vi "CheckConnection.vi"(8 "error in (no error)":errorcluster, 11 "VISA Refnum in":refnum<visa-resource-name>) -> (0 "error out":errorcluster, 3 "Communication succeded?":bool)   [LabVIEW 2018]
doc: "Sends Set Target Command to Maestro channel 5 with control value and checks if value returned after sending Get Position command will correspond, if it does then communication succeded."
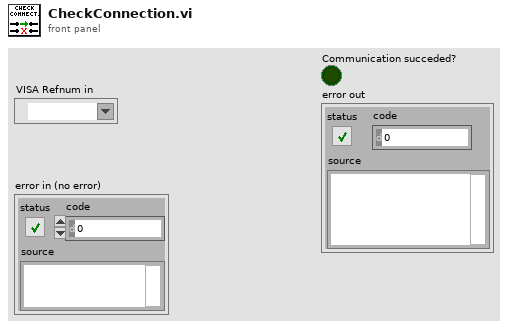
[diagram p1: front panel]
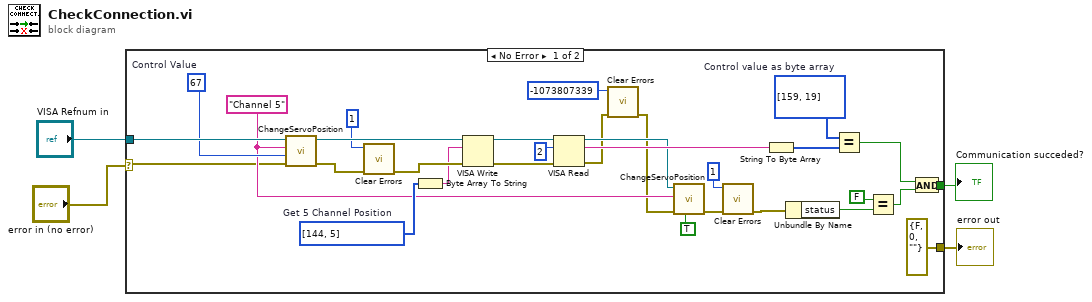
[diagram p0: block diagram]
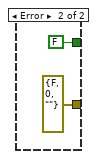
[diagram p2: hidden frame]
diagram:
  n1 = case shown="No Error" "error in (no error)" {
    selector: "error in (no error)" -> [w6 _]
    tunnel: [w32 FALSE] -> w4
    tunnel: "VISA Refnum in" -> [w29 _]
    tunnel: [errorcluster {"status"=FALSE, "code"=0, "source"=""} ("error out") errorcluster {"status"=FALSE, "code"=0, "source"=""} ("error out")] -> w2
    frame No Error {
      w21 = u8[] [144, 5]  # Get 5 Channel Position
      w15 = "Channel 5" ("Label.Text")
      w28 = i16 67  # Control Value
      w16 = u8[] [159, 19]  # Control value as byte array
      n2 = call "ChangeServoPosition.vi"("error in (no error)"=w6, "Value"=w28, "Label.Text"=w15, "VISA Refnum in"=w29) -> ("error out"=w27:errorcluster, "VISA resource name out"=w26:refnum<visa-resource-name>)  [unwired: 6 in]
      n3 = call <vilib>:"Clear Errors.vi"("error in (no error)"=w27, "specific error code to clear (0: all)"=1) -> ("error out"=w25:errorcluster)  [unwired: 4 in, 1 out]
      n4 = Byte Array To String(unsigned byte array=w21) -> (string=w22:string)
      n5 = VISA Write(VISA resource name=w26, write buffer=w22, error in (no error)=w25) -> (VISA resource name out=w24:refnum<visa-resource-name>, error out=w23:errorcluster)  [unwired: 1 out]
      n6 = VISA Read(VISA resource name=w24, byte count=u32 2, error in (no error)=w23) -> (VISA resource name out=w14:refnum<visa-resource-name>, read buffer=w34:string, error out=w8:errorcluster)  [unwired: 1 out]
      n7 = call <vilib>:"Clear Errors.vi"("error in (no error)"=w8, "specific error code to clear (0: all)"=-1073807339) -> ("error out"=w7:errorcluster)  [unwired: 4 in, 1 out]
      n8 = call "ChangeServoPosition.vi"("Close communication"=TRUE, "error in (no error)"=w7, "Label.Text"=w15, "VISA Refnum in"=w14) -> ("error out"=w12:errorcluster)  [unwired: 6 in, 1 out]
      n9 = call <vilib>:"Clear Errors.vi"("error in (no error)"=w12, "specific error code to clear (0: all)"=1) -> ("error out"=w11:errorcluster)  [unwired: 4 in, 1 out]
      n10 = String To Byte Array(string=w34) -> (unsigned byte array=w17:u8[])
      n11 = Unbundle By Name(w11) -> ("status"=w31:bool)
      n12 = Equal?(x=w16, y=w17) -> (x = y?=w19:bool)
      n13 = Equal?(x=FALSE, y=w31) -> (x = y?=w18:bool)
      n14 = And(x=w19, y=w18) -> (x .and. y?=w32:bool)
    }
    frame Error {
    }
  }
  "Communication succeded?" <- w4
  "error out" <- w2
